vi "GetChosenDevice.vi"(11 "Index":i32) -> (3 "Device Out":refnum<class "Device.lvclass">)   [LabVIEW 2013]
uses:
  Device/Device.lvclass
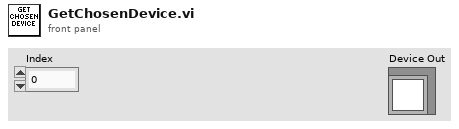
[diagram p1: front panel]
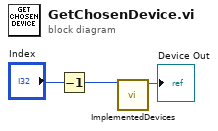
[diagram p0: block diagram]
diagram:
  n1 = Decrement(x="Index") -> (x-1=w3:i32)
  n2 = call "ImplementedDevices.vi"("Index"=w3) -> ("Device Out"=→"Device Out":refnum<class "Device.lvclass">)  [unwired: 8 in, 2 out]
